vi "Get Channel Properties.vi"(10 "Log Properties":bool, 11 "TDMS Channel Info":T1) -> (3 "Property String Out":string[](array[string]))   [LabVIEW 2022 SP3]
uses:
  CSV Export.lvclass
panel:
  in  "Date Format":string
  in  "Digits of Precision":i32
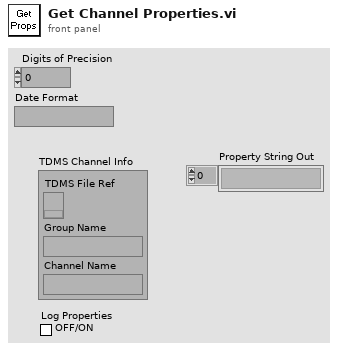
[diagram p1: front panel]
types:
  T1 = cluster{"TDMS File Ref":refnum<k34>, "Group Name":string, "Channel Name":string}
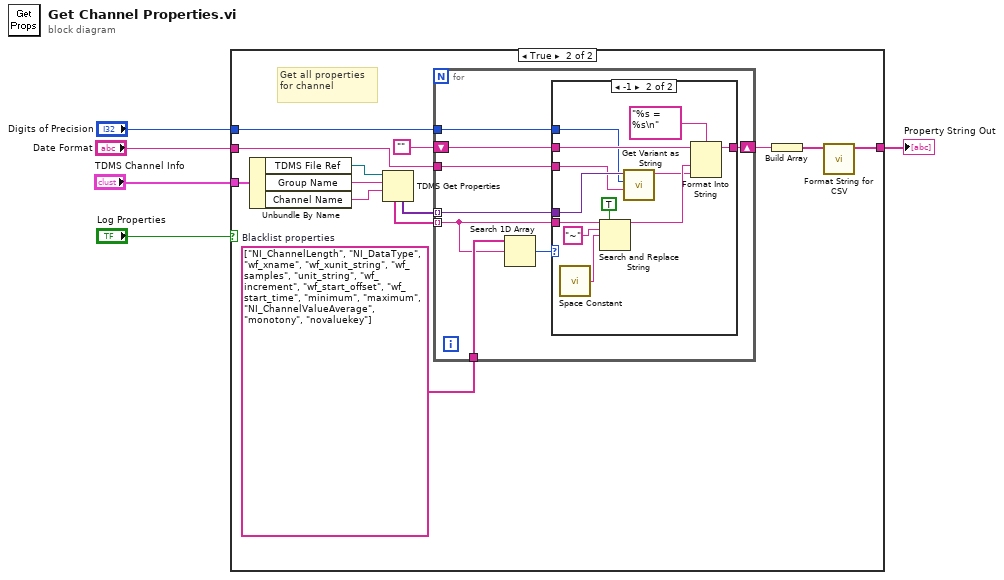
[diagram p0: block diagram]
diagram:
  n1 = case shown="True" "Log Properties" {
    tunnel: "TDMS Channel Info" -> [_ w18]
    tunnel: [_ w6] -> w3
    tunnel: "Date Format" -> [_ w9]
    tunnel: "Digits of Precision" -> [_ w8]
    frame False {
    }
    frame True {
      w12 = string[] ["NI_ChannelLength", "NI_DataType", "wf_xname", "wf_xunit_string", "wf_samples", "unit_string", "wf_increment", "wf_start_offset", "wf_start_time", "minimum", "maximum", "NI_ChannelValueAverage", "monotony", "novaluekey"]  # Blacklist properties
      # "Get all properties for channel"
      n2 = Unbundle By Name(w18) -> ("TDMS File Ref"=w17:refnum<k34>, "Group Name"=w16:string, "Channel Name"=w15:string)
      n3 = TDMS Get Properties(9:w15, 10:w16, 11:w17) -> (4:w13:variant[], 6:w14:string[])  [unwired: 3 in, 4 out]
      n4 = for {
        tunnel: w14 -> [w24] mode=indexing
        tunnel: w13 -> [w23] mode=indexing
        tunnel: w12 -> [w26]
        shift-right: [w21] -> w10
        shift-left: "" -> [w22]
        tunnel: w9 -> [w20]
        tunnel: w8 -> [w19]
        n5 = Search 1D Array(1D array=w26, element=w24) -> (index of element=w25:i32)  [unwired: 1 in]
        n6 = case shown="-1" w25 {
          tunnel: w24 -> [_ w39]
          tunnel: w23 -> [_ w31]
          tunnel: w22 -> [w27 w36]
          tunnel: [w27 w34] -> w21
          tunnel: w20 -> [_ w29]
          tunnel: w19 -> [_ w28]
          frame 0, Default {
          }
          frame -1 {
            n7 = call <vilib>:"Space Constant.vi"() -> ("String"=w37:string)
            n8 = Search and Replace String(replace all?=TRUE ("replace all? (F)"), input string=w39, search string="~", replace string=w37) -> (result string=w32:string)  [unwired: 4 in, 3 out]
            n9 = call "Get Variant as String.vi"("time format string (%c)"=w29, "Digits of Precision"=w28, "Variant"=w31) -> ("Variant Value as String"=w30:string)  [unwired: 8 in]
            n10 = Format Into String(format string="%s = %s\n", initial string=w36, w32, w30) -> (resulting string=w34:string)  [unwired: 1 in, 1 out]
          }
        }
      }
      n11 = Build Array(w10) -> (w7:string[])
      n12 = call "Format String for CSV.vi"("Row Data"=w7) -> ("CSV Formatted strings"=w6:string[])  [unwired: 10 in]
    }
  }
  "Property String Out" <- w3
